vi "Read Unicode Text from File - Display as Unicode.vi"() -> ()   [LabVIEW 2009]
panel:
  out "File Contents (Hex)":string
  out "File Contents (Unicode Display)":string
  out "File Contents (ASCII Display)":string
  out "String":string caption="Greeting"
  # "Unicode String Indicator"
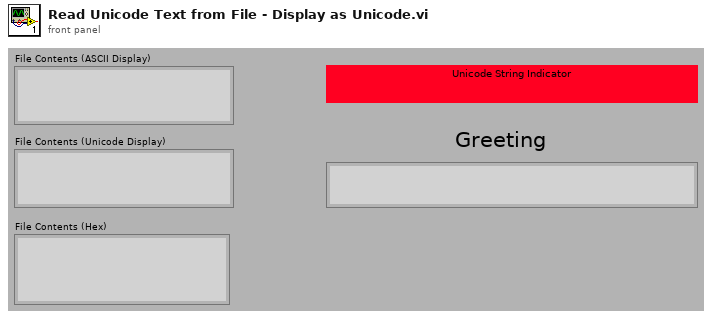
[diagram p1: front panel]
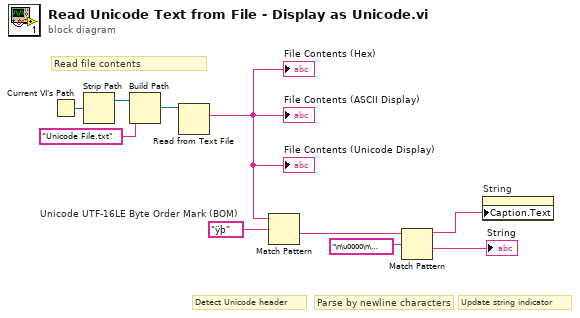
[diagram p0: block diagram]
diagram:
  w6 = "ÿþ"  # Unicode UTF-16LE Byte Order Mark (BOM)
  # "Update string indicator"
  # "Parse by newline characters"
  # "Detect Unicode header"
  # "Read file contents"
  n1 = Current VI's Path() -> (path=w10:path)
  n2 = Strip Path(path=w10) -> (stripped path=w9:path)  [unwired: 1 out]
  n3 = Build Path(base path=w9, name or relative path="Unicode File.txt") -> (appended path=w7:path)
  n4 = Read from Text File(file (use dialog)=w7) -> (text=w3:string)  [unwired: 3 in, 3 out]
  "File Contents (ASCII Display)" <- w3
  "File Contents (Unicode Display)" <- w3
  "File Contents (Hex)" <- w3
  n5 = Match Pattern(string=w3, regular expression=w6) -> (after substring=w5:string)  [unwired: 1 in, 3 out]
  n6 = Match Pattern(string=w5, regular expression="\n\u0000\n\u0000") -> (before substring=w1:string, after substring=→"String":string)  [unwired: 1 in, 2 out]
  n7 = property on="String" class="Str"("Caption.Text"=w1) -> ()  [unwired: 2 in, 2 out]
